vi "applyDelays.vi"(8 "error in (no error)":errorcluster, 10 "globalDelay":dbl, 11 "ScriptEvent in":refnum<class "ScriptEvent.lvclass">) -> (0 "error out":errorcluster, 2 "globalDelay out":dbl, 3 "ScriptEvent out":refnum<class "ScriptEvent.lvclass">)   [LabVIEW 2011, in "Tools.lvlib" / "Scripting.lvlib" / "ScriptEvent.lvclass"]
uses:
  ScriptEvent.lvclass
  ScriptEvent.lvclass/ScriptEvent.ctl
  DatabaseHelpers/Database Objects/Channel/DigitalChannel/DigitalChannel.lvclass
  DatabaseHelpers/Database Objects/Channel/Channel.lvclass
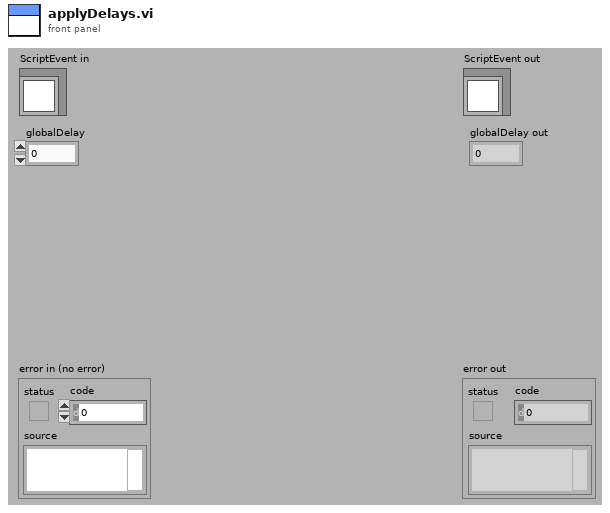
[diagram p1: front panel]
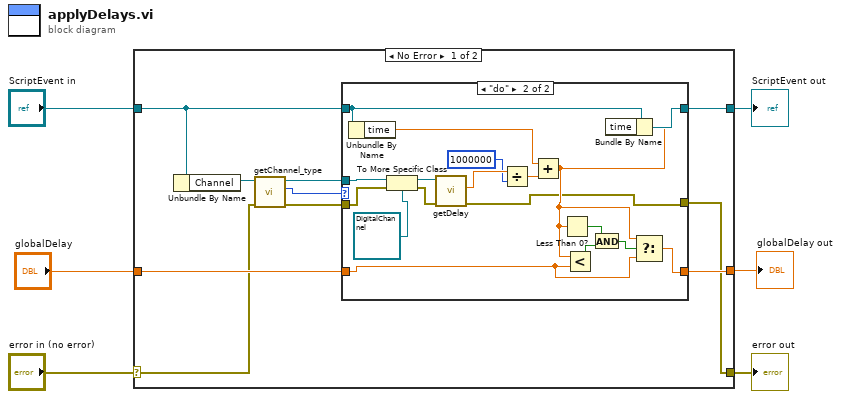
[diagram p0: block diagram]
diagram:
  n1 = case shown="No Error" "error in (no error)" {
    selector: "error in (no error)" -> [w10 w39]
    tunnel: [w7 w39] -> w5
    tunnel: [w8 w38] -> w3
    tunnel: "ScriptEvent in" -> [w9 w38]
    tunnel: "globalDelay" -> [w12 _]
    tunnel: [w11 _] -> w1
    frame No Error {
      n2 = Unbundle By Name(w9) -> ("Channel"=w16:refnum<class "Channel.lvclass">)
      n3 = call "getChannel_type.vi"("error in (no error)"=w10, "Channel.lvclass in"=w16) -> ("error out"=w13:errorcluster, "channel_type"=w15:enum16{"ao", "do", "ai", "di", "rf"}, "Channel.lvclass out"=w14:refnum<class "Channel.lvclass">)  [unwired: 7 in]
      n4 = case shown="\"do\"" w15 {
        tunnel: w14 -> [_ w36]
        tunnel: w13 -> [w17 w37]
        tunnel: w12 -> [w19 w25]
        tunnel: [w19 w24] -> w11
        tunnel: w9 -> [w18 w31]
        tunnel: [w18 w30] -> w8
        tunnel: [w17 w23] -> w7
        frame Default {
        }
        frame "do" {
          n5 = Unbundle By Name(w31) -> ("time"=w32:dbl)
          n6 = To More Specific Class(target class=refnum<class "DigitalChannel.lvclass"> refnum ("Tools.lvlib:DatabaseHelpers.lvlib:DigitalChannel.lvclass"), reference=w36, error in=w37) -> (specific class reference=w33:refnum<class "DigitalChannel.lvclass">, error out=w34:errorcluster)
          n7 = call "getDelay.vi"("error in (no error)"=w34, "DigitalChannel.lvclass in"=w33) -> ("error out"=w23:errorcluster, "delay"=w21:dbl)  [unwired: 7 in, 1 out]
          n8 = Divide(x=w21, y=1000000) -> (x/y=w22:dbl)
          n9 = Add(x=w32, y=w22) -> (x+y=w26:dbl)
          n10 = Less Than 0?(x=w26) -> (x < 0?=w29:bool)
          n11 = Less?(x=w26, y=w25) -> (x < y?=w28:bool)
          n12 = And(x=w29, y=w28) -> (x .and. y?=w27:bool)
          n13 = Bundle By Name(cluster=w31, "time"=w26) -> (w30:refnum<class "ScriptEvent.lvclass">)
          n14 = Select(t=w26, s=w27, f=w25) -> (s? t:f=w24:dbl)
        }
      }
    }
    frame Error {
    }
  }
  "error out" <- w5
  "ScriptEvent out" <- w3
  "globalDelay out" <- w1
